vi "WriteEvent.vi"(3 "Evt name":string="Event Data", 4 "Digitizer Data":i16[][](array[numeric]), 5 "QDC Data":i16[](array[numeric]), 6 "TDC Data":i16[](array[numeric]), 7 "Scaler Data":u32[](array[numeric]), 8 "error in":errorcluster, 9 "Trigger Bits (as U64)":u64, 10 "Temperature":sgl, 11 "file ref in":T1 format="%.0x") -> (0 "error out":errorcluster)   [LabVIEW 2014]
uses:
  <vilib>/addons/h5labview2/base/hid_t.ctl
  DatasetNames.vi
  <vilib>/addons/h5labview2/base/lib_path.vi
  <vilib>/addons/h5labview2/base/H5Equery.vi
  <vilib>/addons/h5labview2/dataset/H5Dwrite.llb/H5Dwrite.xnode
  <vilib>/addons/h5labview2/group/H5G.lvlib
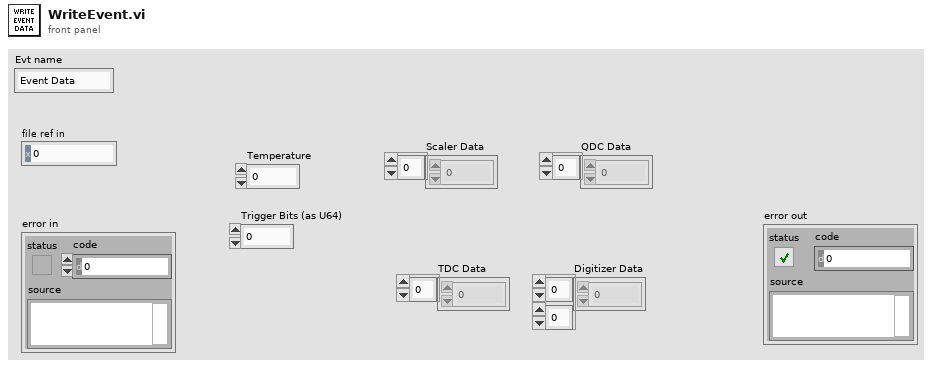
[diagram p1: front panel]
types:
  T1 = typedef "hid_t.ctl" = i32
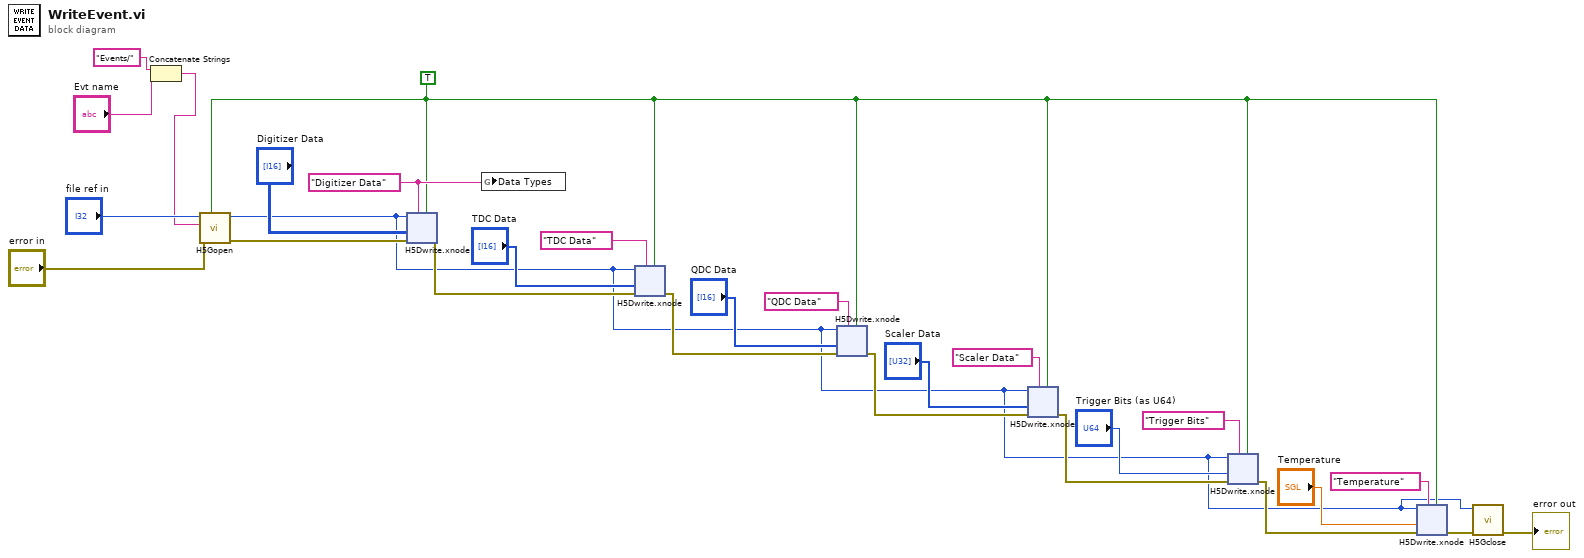
[diagram p0: block diagram]
diagram:
  w7 = TRUE ("replace? (F)")
  w24 = "Digitizer Data" ("Combo Box")
  n1 = Concatenate Strings("Events/", "Evt name") -> (w2:string)
  n2 = call <vilib>:"H5Gopen.vi"("create? (F)"=w7, "error in (no error)"="error in", "name"=w2, "ref in"="file ref in") -> ("error out"=w23:errorcluster, "group out"=w5:T1)  [unwired: 6 in]
  n3 = xnode "H5Dwrite.xnode"("replace? (F)"=w7, "dataset name"=w24, "error in (no error)"=w23, "data"="Digitizer Data", "ref in"=w5) -> ("error out"=w20:errorcluster)  [unwired: 2 in, 2 out]
  n4 = global write "DatasetNames.vi" "Data Types"(w24) -> ()
  n5 = xnode "H5Dwrite.xnode"("replace? (F)"=w7, "dataset name"="TDC Data" ("Combo Box"), "error in (no error)"=w20, "data"="TDC Data", "ref in"=w5) -> ("error out"=w19:errorcluster)  [unwired: 2 in, 2 out]
  n6 = xnode "H5Dwrite.xnode"("replace? (F)"=w7, "dataset name"="QDC Data" ("Combo Box"), "error in (no error)"=w19, "data"="QDC Data", "ref in"=w5) -> ("error out"=w16:errorcluster)  [unwired: 2 in, 2 out]
  n7 = xnode "H5Dwrite.xnode"("replace? (F)"=w7, "dataset name"="Scaler Data" ("Combo Box"), "error in (no error)"=w16, "data"="Scaler Data", "ref in"=w5) -> ("error out"=w13:errorcluster)  [unwired: 2 in, 2 out]
  n8 = xnode "H5Dwrite.xnode"("replace? (F)"=w7, "dataset name"="Trigger Bits" ("Combo Box"), "error in (no error)"=w13, "data"="Trigger Bits (as U64)", "ref in"=w5) -> ("error out"=w10:errorcluster)  [unwired: 2 in, 2 out]
  n9 = xnode "H5Dwrite.xnode"("replace? (F)"=w7, "dataset name"="Temperature" ("Combo Box"), "error in (no error)"=w10, "data"="Temperature", "ref in"=w5) -> ("error out"=w4:errorcluster)  [unwired: 2 in, 2 out]
  n10 = call <vilib>:"H5Gclose.vi"("error in (no error)"=w4, "group in"=w5) -> ("error out"=→"error out":errorcluster)  [unwired: 9 in]
